vi "FPGA Target Approach Retraction2(2).vi"() -> ()   [LabVIEW 2012]
uses:
  <vilib>/rvi/Emulation/niFpgaSctlEmulationGetInTimedLoop.vi
  <vilib>/rvi/Emulation/niFpgaSctlEmulationGlobalWrite.vi
  <vilib>/rvi/interface/RandomDataEmulation/nirviRandomDataFPGAFIFO.vi
  <vilib>/rvi/interface/RandomDataEmulation/niFpgaRandomDataHandleErrors.vi
  <vilib>/rvi/eio/common/nirviEmuTemplateMethod_errors.vi
  <vilib>/rvi/DataTransferAndStorage/Container/XNode/niFpgaContainer.xnode
  <vilib>/rvi/interface/RandomDataEmulation/nirviRandomDataFpgaReadWriteTemplate.vi
  <vilib>/eio/EIONode/EIONode.xnode
  <vilib>/rvi/Analysis/measure/butterworth/XNode/niFpgaButterworthFilter.xnode
panel:
  in  "Manual Approach Start":bool
  in  "Automated FPGA Start":bool
  out "Counter Output 2":fxp<+/-,16,16>
  out "Bit/us":fxp<+/-,64,41>
  in  "Bit/nm converter":fxp<+,26,2>
  in  "Fast Approach Speed":i16
  out "Multiplier":i16
  out "Numeric 2":i16
  out "Numeric":i16
  out "Ticks":i16
  out "Ticks":i16
  in  "Data Acquisition Rate":i16
  out "HV/10":i16
  out "Tuning Fork Signal":fxp<+/-,24,17>
  out "FPGA Output Voltage":fxp<+/-,64,32>
  out "Z Fine Indicator":fxp<+/-,40,30>
  out "Counter Indicator":i32
  in  "Z Fine Output":fxp<+/-,40,30>
  in  "Counter Output":i32
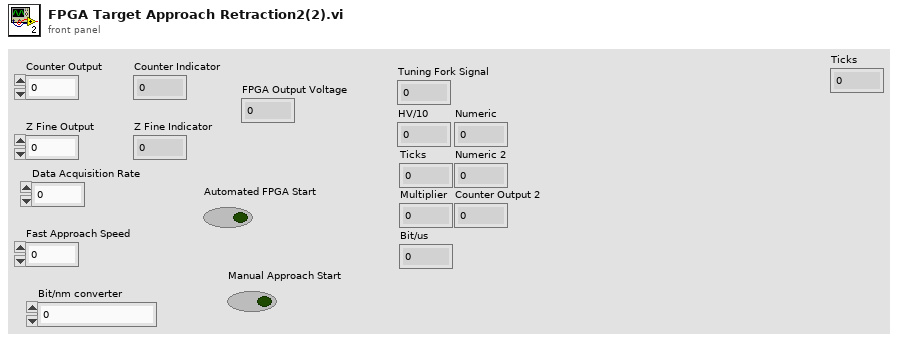
[diagram p1: front panel]
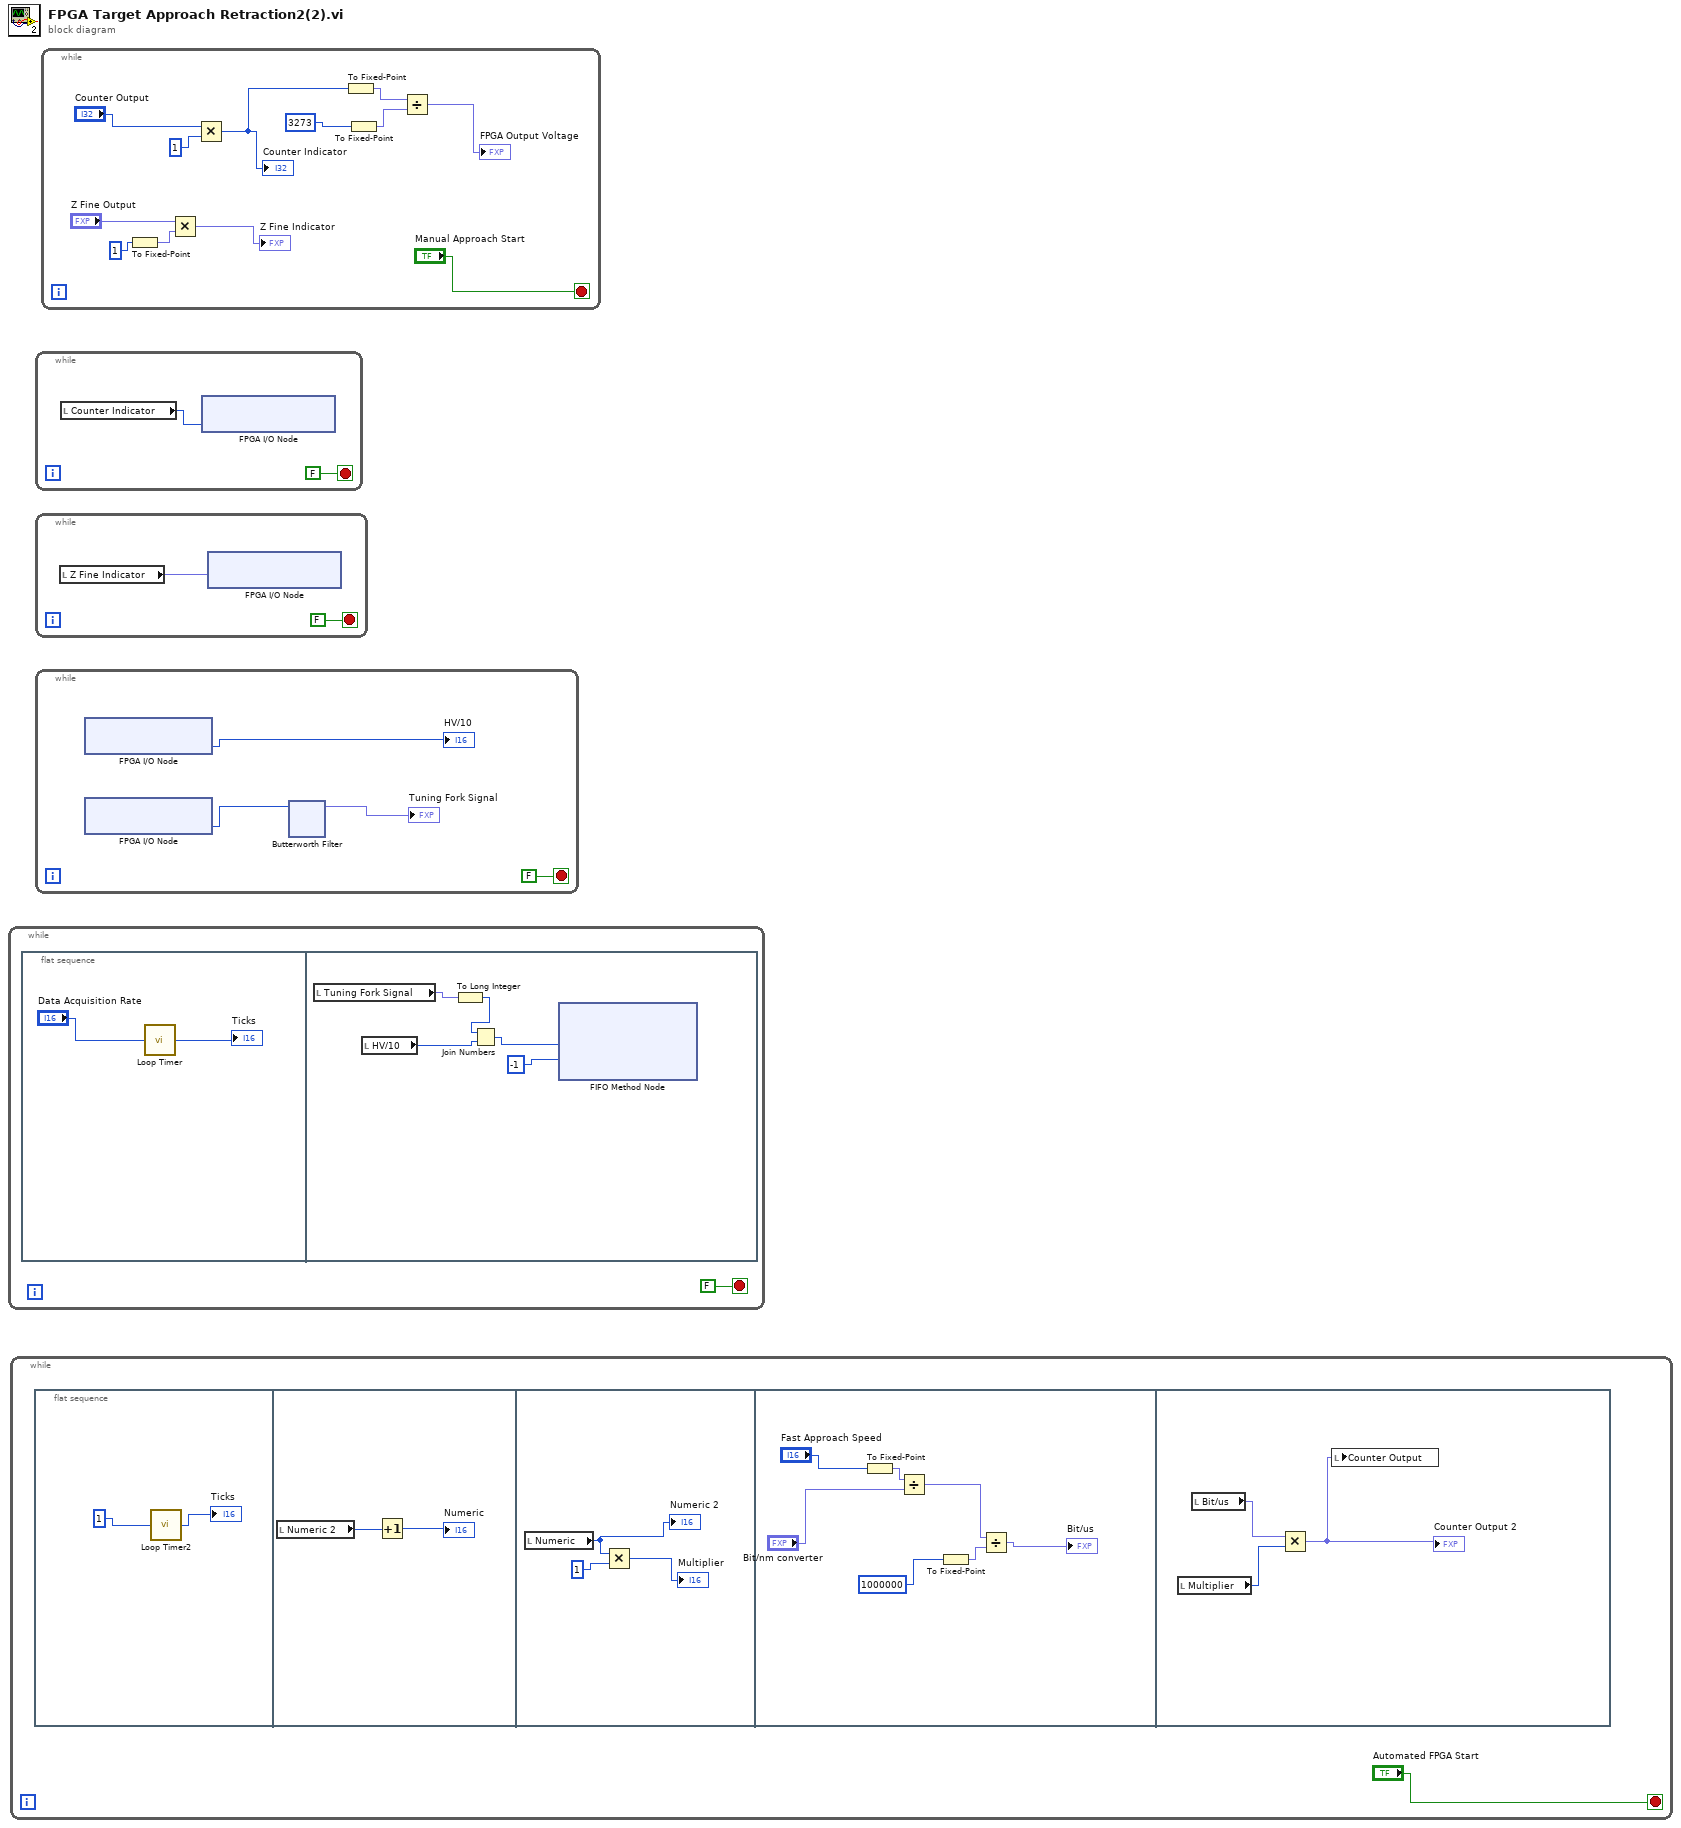
[diagram p0: block diagram]
diagram:
  n1 = while {
    stop <- FALSE stop-if-true
    n2 = flat-sequence {
      frame #0 {
        n3 = call "Loop Timer"("Count(uSec)"="Data Acquisition Rate") -> ("Tick Count(uSec)"=→"Ticks":u32)
      }
      frame #1 {
        n4 = local read "Tuning Fork Signal"() -> (w7:fxp<+/-,24,17>)
        n5 = local read "HV/10"() -> (w8:i16)
        n6 = To Long Integer(number=w7) -> (32bit integer=w6:i32)
        n7 = Join Numbers(hi=w6, lo=w8) -> ((hi.lo)=w5:u64)
        n8 = xnode ("FIFO Method Node")("Element"=w5, "Timeout"=i16 -1) -> ()  [unwired: 1 in, 2 out]
      }
    }
  }
  n9 = while {
    stop <- "Automated FPGA Start" stop-if-true
    n10 = flat-sequence {
      frame #0 {
        n11 = call "Loop Timer2"("Count(uSec)"=i16 1) -> ("Tick Count(uSec)"=→"Ticks":u32)
      }
      frame #1 {
        n12 = local read "Numeric 2"() -> (w12:i16)
        n13 = Increment(x=w12) -> (x+1=→"Numeric":i16)
      }
      frame #2 {
        n14 = local read "Numeric"() -> (w15:i16)
        "Numeric 2" <- w15
        n15 = Multiply(x=w15, y=i16 1) -> (x*y=→"Multiplier":i16)
      }
      frame #3 {
        n16 = To Fixed-Point(number="Fast Approach Speed") -> (fixed-point=w22:fxp<+/-,16,16>)  [unwired: 1 in]
        n17 = Divide(x=w22, y="Bit/nm converter") -> (x/y=w18:fxp<+/-,42,40>)
        n18 = To Fixed-Point(number=1000000) -> (fixed-point=w20:fxp<+/-,32,32>)  [unwired: 1 in]
        n19 = Divide(x=w18, y=w20) -> (x/y=→"Bit/us":fxp<+/-,64,41>)
      }
      frame #4 {
        n20 = local read "Multiplier"() -> (w26:i16)
        n21 = local read "Bit/us"() -> (w25:fxp<+/-,64,41>)
        n22 = Multiply(x=w25, y=w26) -> (x*y=w24:fxp<+/-,64,57>)
        "Counter Output 2" <- w24
        n23 = local write "Counter Output"(w24) -> ()
      }
    }
  }
  n24 = while {
    stop <- FALSE stop-if-true
    n25 = local read "Counter Indicator"() -> (w27:i32)
    n26 = xnode "FPGA I/O Node"("Connector0/AO7"=w27) -> ()  [unwired: 1 in, 1 out]
  }
  n27 = while {
    stop <- FALSE stop-if-true
    n28 = local read "Z Fine Indicator"() -> (w29:fxp<+/-,40,30>)
    n29 = xnode "FPGA I/O Node"("Connector0/AO2"=w29) -> ()  [unwired: 1 in, 1 out]
  }
  n30 = while {
    stop <- FALSE stop-if-true
    n31 = xnode "FPGA I/O Node"() -> ("Connector0/AI6"=→"HV/10":i16)  [unwired: 1 in, 1 out]
    n32 = xnode "FPGA I/O Node"() -> ("Connector0/AI7"=w33:i16)  [unwired: 1 in, 1 out]
    n33 = xnode "Butterworth Filter"("input data"=w33) -> ("output data"=→"Tuning Fork Signal":fxp<+/-,20,20>)  [unwired: 2 in]
  }
  n34 = while {
    stop <- "Manual Approach Start" stop-if-true
    n35 = To Fixed-Point(number=1) -> (fixed-point=w49:fxp<+/-,32,32>)  [unwired: 1 in]
    n36 = Multiply(x="Z Fine Output", y=w49) -> (x*y=→"Z Fine Indicator":fxp<+/-,64,62>)
    n37 = Multiply(x="Counter Output", y=1) -> (x*y=w47:i32)
    "Counter Indicator" <- w47
    n38 = To Fixed-Point(number=w47) -> (fixed-point=w46:fxp<+/-,32,32>)  [unwired: 1 in]
    n39 = To Fixed-Point(number=3273) -> (fixed-point=w45:fxp<+/-,32,32>)  [unwired: 1 in]
    n40 = Divide(x=w46, y=w45) -> (x/y=→"FPGA Output Voltage":fxp<+/-,64,33>)
  }
